vi "Format Save Path.vi"(10 "Filename":string, 11 "DCIMG Path":path) -> (3 "appended path":path)   [LabVIEW 2015, in "Camera.lvlib"]
uses:
  Camera.lvlib
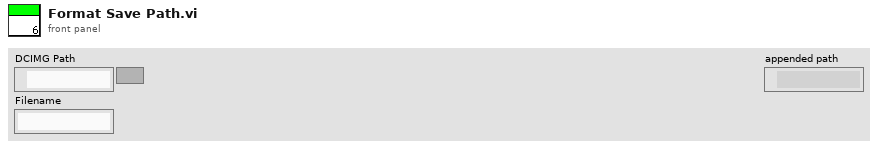
[diagram p1: front panel]
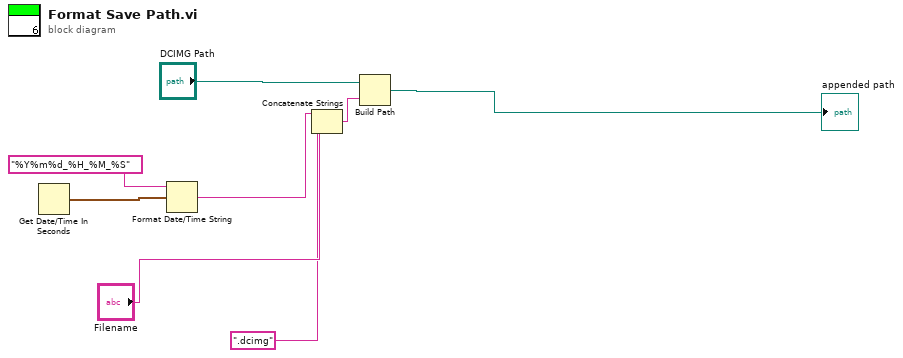
[diagram p0: block diagram]
diagram:
  n1 = Get Date/Time In Seconds() -> (seconds since 1Jan1904=w3:timestamp)
  n2 = Format Date/Time String(time format string (%c)="%Y%m%d_%H_%M_%S", seconds (now)=w3) -> (date/time string=w1:string)  [unwired: 1 in]
  n3 = Concatenate Strings(w1, "Filename", ".dcimg" ("Filename")) -> (w6:string)
  n4 = Build Path(base path="DCIMG Path", name or relative path=w6) -> (appended path=→"appended path":path)
